vi "Get_Element.vi"(1 "Search for string":string, 2 "Det. list":dbl[](array[numeric]), 3 "Meas. Data":dbl[](array[numeric])) -> (0 "Output":u32)   [LabVIEW 2010]
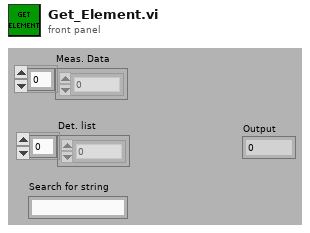
[diagram p1: front panel]
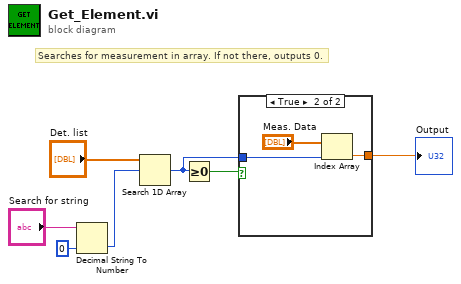
[diagram p0: block diagram]
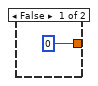
[diagram p2: hidden frame]
diagram:
  # "Searches for measurement in array. If not there, outputs 0."
  n1 = Decimal String To Number(string="Search for string", default (0L)=i8 0) -> (number=w4:i8)  [unwired: 1 in, 1 out]
  n2 = Search 1D Array(1D array="Det. list", element=w4) -> (index of element=w2:i32)  [unwired: 1 in]
  n3 = Greater Or Equal To 0?(x=w2) -> (x >= 0?=w3:bool)
  n4 = case shown="True" w3 {
    tunnel: w2 -> [_ w10]
    tunnel: [0 w9] -> w1
    frame False {
    }
    frame True {
      n5 = Index Array(array="Meas. Data", index=w10) -> (element=w9:dbl)
    }
  }
  "Output" <- w1
